vi "Stop Core.vi"(10 "final error code":i32, 11 "UI_Actor in":refnum<class "UI_Actor.lvclass">) -> (3 "UI_Actor out":refnum<class "UI_Actor.lvclass">)   [LabVIEW 2020, in "UI_Actor.lvlib" / "UI_Actor.lvclass"]
doc: "(<B>Filename</B>: Actor Framework.lvlib:Actor.lvclass:Stop Core.vi)\n\nDefines what the actor does before it stops. Use the <B>final error code</B> input to determine whether the actor shut down in response to an error.\n\nBy default, this method does nothing. A descendant class may override it to define behavior, such as shutting down any processes the actor initiated in its override of the Actor Core method."
uses:
  UI_Actor.lvclass
  ctl_UE_Msg.ctl
  UI_Actor.lvclass/UI_Actor.ctl
  support/Actor Framework.lvlibp/1abvi3w/vi.lib/ActorFramework/Actor/Actor.lvclass
panel:
  out "error out 2":errorcluster
  out "error out":errorcluster
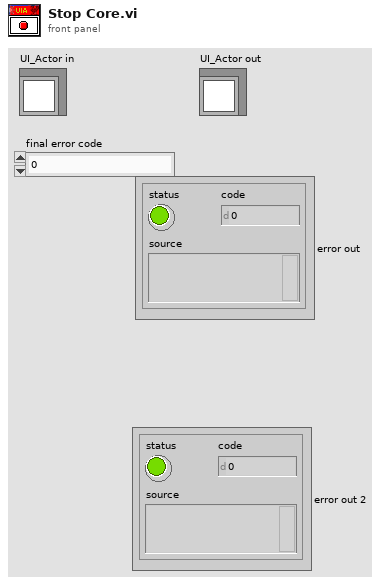
[diagram p1: front panel]
types:
  T1 = typedef "UI_Actor.lvlib/UI_Actor.lvclass/ctl_UE_Msg.ctl" = cluster{"Cmd":string, "Payload":string}
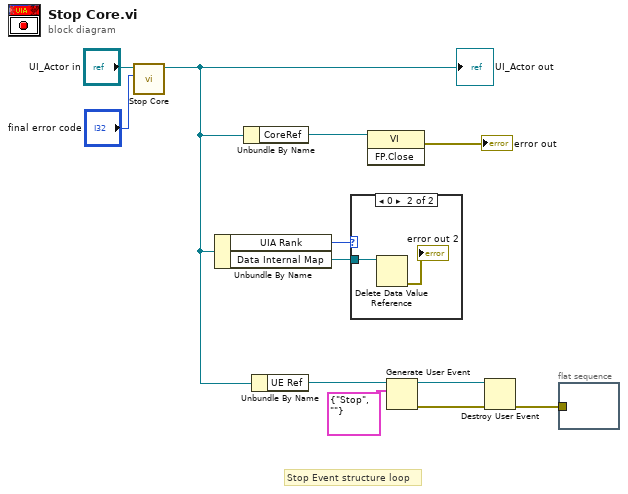
[diagram p0: block diagram]
diagram:
  # "Stop Event structure loop"
  n1 = call-parent "Stop Core.vi"("final error code"="final error code", "Actor in"="UI_Actor in") -> ("Actor out"=w6:refnum<class "UI_Actor.lvclass">)  [unwired: 9 in]
  "UI_Actor out" <- w6
  n2 = Unbundle By Name(w6) -> ("UIA Rank"=w8:i32, "Data Internal Map"=w7:refnum<data-value>)
  n3 = Unbundle By Name(w6) -> ("CoreRef"=w10:refnum<vi>)
  n4 = Unbundle By Name(w6) -> ("UE Ref"=w4:refnum<user-event>)
  n5 = case shown="0" w8 {
    tunnel: w7 -> [_ w14]
    frame Default {
    }
    frame 0 {
      n6 = Delete Data Value Reference(data value reference=w14) -> (error out=→"error out 2":errorcluster)  [unwired: 1 in, 1 out]
    }
  }
  n7 = invoke class="VI" method="FP.Close"(reference=w10) -> (error out=→"error out":errorcluster)  [unwired: 2 in, 2 out]
  n8 = Generate User Event(user event=w4, event data cluster=T1 {"Cmd"="Stop", "Payload"=""} ("event data")) -> (user event out=w3:refnum<user-event>, error out=w2:errorcluster)  [unwired: 2 in]
  n9 = Destroy User Event(user event=w3, error in=w2) -> (error out=w5:errorcluster)
  n10 = flat-sequence {
    tunnel: w5 -> [_]
    frame #0 {
    }
  }
